vi "UpdateBugTrail.vi"(11 "Start Goal Data":T1) -> (3 "Start Goal Data out":T1)   [LabVIEW 2013]
uses:
  Bug_StartGoalData.ctl
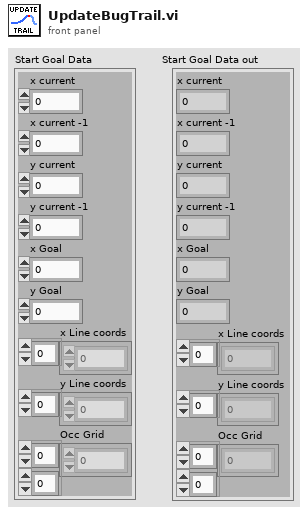
[diagram p1: front panel]
types:
  T1 = typedef "Bug_StartGoalData.ctl" = cluster{"x current":i32, "x current -1":i32, "y current":i32, "y current -1":i32, "x Goal":i32, "y Goal":i32, "x Line coords":i32[], "y Line coords":i32[], "Occ Grid":dbl[][]}
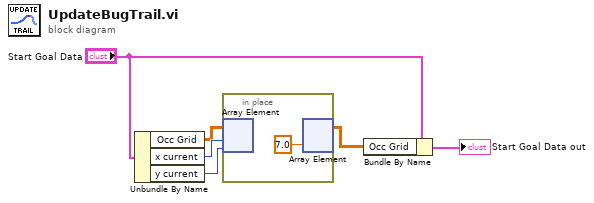
[diagram p0: block diagram]
diagram:
  n1 = Unbundle By Name("Start Goal Data") -> ("Occ Grid"=w4:dbl[][], "x current"=w6:i32, "y current"=w5:i32)
  n2 = in-place {
    n3 = in-place-array #1(w4, w6, w5) -> ()  [unwired: 1 out]
    n4 = in-place-array #1(7.0) -> (w3:dbl[][])  [unwired: 2 out]
  }
  n5 = Bundle By Name(cluster="Start Goal Data", "Occ Grid"=w3) -> (→"Start Goal Data out":T1)
